vi "List Devices.vi"(8 "error in (no error)":errorcluster, 11 "Spark Reference In":T1) -> (0 "error out":errorcluster, 2 "Devices JSON":T4, 3 "Spark Reference Out":T1)   [LabVIEW 2014, in "Spark API.lvlib"]
doc: "Lists all the Spark devices registered to a given account, along with their current online/offline status."
uses:
  Spark API.lvlib
  Controls/Devices Query JSON.ctl
  Controls/Spark Reference.ctl
  <vilib>/httpClient/ClientHandle.ctl
  Controls/Device Query JSON.ctl
  <vilib>/httpClient/LabVIEWHTTPClient.lvlib
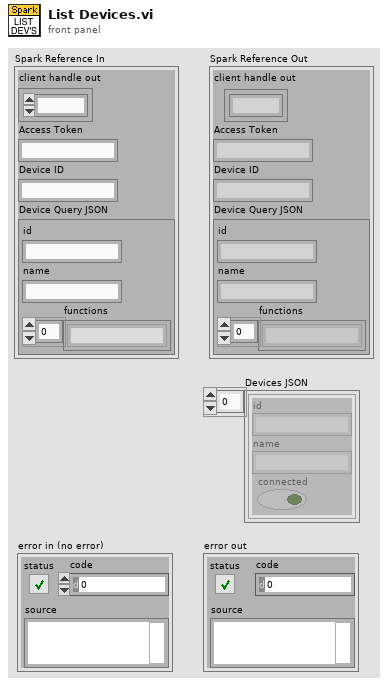
[diagram p1: front panel]
types:
  T1 = typedef "Spark API.lvlib/Spark Reference.ctl" = cluster{"client handle out":T2, "Access Token":string, "Device ID":string, "Device Query JSON":T3}
  T2 = typedef "LabVIEWHTTPClient.lvlib/ClientHandle.ctl" = refnum<k1>
  T3 = typedef "Spark API.lvlib/Device Query JSON.ctl" = cluster{"id":string, "name":string, "functions":string[]}
  T4 = typedef "Spark API.lvlib/Devices Query JSON.ctl" = cluster{"id":string, "name":string, "connected":bool}[]
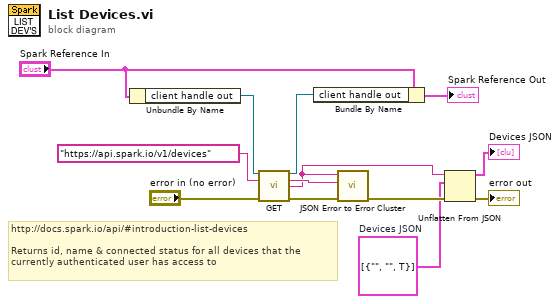
[diagram p0: block diagram]
diagram:
  w5 = T4 [{"id"="", "name"="", "connected"=TRUE}]  # Devices JSON
  # "http://docs.spark.io/api/#introduction-list-devices\n\nReturns id, name & connected status for all devices that the currently authenticated user has access to"
  n1 = Unbundle By Name("Spark Reference In") -> ("client handle out"=w4:T2)
  n2 = call <vilib>:"GET.vi"("client handle"=w4, "url"="https://api.spark.io/v1/devices", "error in (no error)"="error in (no error)") -> ("client handle out"=w2:T2, "headers"=w11:string, "body"=w10:string, "error out"=w8:errorcluster)  [unwired: 9 in]
  n3 = Bundle By Name(cluster="Spark Reference In", "client handle out"=w2) -> (→"Spark Reference Out":T1)
  n4 = call "JSON Error to Error Cluster.vi"("error in (no error)"=w8, "headers"=w11, "JSON string"=w10) -> ("error out"=w9:errorcluster)  [unwired: 8 in]
  n5 = Unflatten From JSON(JSON string=w10, type and defaults=w5, error in (no error)=w9) -> (value=→"Devices JSON":T4, error out=→"error out":errorcluster)  [unwired: 4 in]
